vi "Update State Name.vi"(8 "error in":errorcluster, 10 "State Name":string, 11 "Series UI Actor in":refnum<class "Series UI Actor.lvclass">) -> (0 "error out":errorcluster, 3 "Series UI Actor out":refnum<class "Series UI Actor.lvclass">)   [LabVIEW 2024, in "Series UI Actor.lvlib" / "Series UI Actor.lvclass"]
uses:
  Series UI Actor.lvclass
  Series UI Actor.lvclass/Series UI Actor.ctl
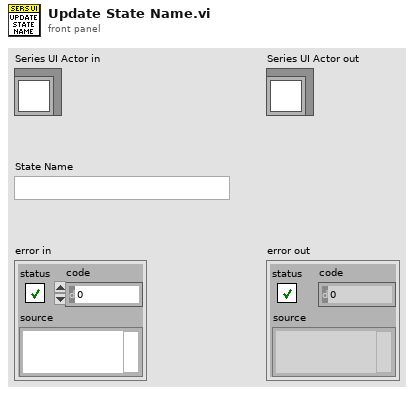
[diagram p1: front panel]
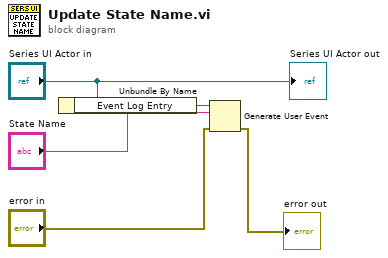
[diagram p0: block diagram]
diagram:
  n1 = Unbundle By Name("Series UI Actor in") -> ("Event Log Entry"=w4:refnum<user-event>)
  n2 = Generate User Event(user event=w4, event data cluster="State Name", error in="error in") -> (error out=→"error out":errorcluster)  [unwired: 1 in, 1 out]
  "Series UI Actor out" <- "Series UI Actor in"
